vi "En-Dis Contrl UI1.vi"(7 "Enable?":bool, 10 "Array":refnum<vi>[](array[refnum])) -> ()   [LabVIEW 2018, in "Testing UI 4.lvlib"]
uses:
  Testing UI 4/Testing UI 4.lvlib
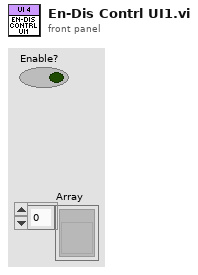
[diagram p1: front panel]
types:
  T1 = enum8{"Enabled", "Disabled", "Disabled and Grayed Out"}
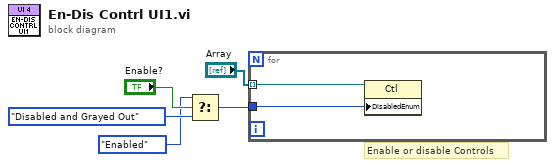
[diagram p0: block diagram]
diagram:
  # "Enable or disable Controls"
  n1 = Select(t=T1."Enabled" ("Disabled"), s="Enable?", f=T1."Disabled and Grayed Out" ("Disabled")) -> (s? t:f=w2:T1)
  n2 = for {
    tunnel: "Array" -> [w7] mode=indexing
    tunnel: w2 -> [w6]
    n3 = property class="Ctl"(reference=w7, "DisabledEnum"=w6) -> ()  [unwired: 1 in, 2 out]
  }
